vi "KeyboardNudge.vi"(0 "WaveformGraph Refnum":refnum<vi>, 1 "Axis Tune Refnum":refnum<vi>, 3 "Char":i16, 4 "Position (mm) Refnum":refnum<vi>, 5 "Ignore Key Down":bool, 6 "VKey":T2, 7 "PlatMods":T7, 10 "Daxsonics Settings":refnum<vi>, 11 "Pulser":T1, 12 "Inc. Step Size (mm)":dbl=0.5, 13 "Motion Settings":T3={"No Motion?"=FALSE, "Motion System"=enum."MM3000", "Motion Bd ID"=0, "Motion Profile"="", "# Axis"=0, "Reverse Z axis?"=FALSE, "SMAC Axis"=0, "scan pair"=enum."y-(x) scan", "RT fps"=0.0, "Steps per mm"=[], "Motor Parameters"={"velocity ct/s"=[], "accel ct/s^2"=[]}, "One Way Scan"=FALSE, "Reverse One Way Scan"=FALSE, "Global Position (mm)"=[], "Plane"=0, "Distance between\nscan lines (um)"=0.0, "Distance between\nscan planes (um)"=0.0, "number of scan planes"=0, "Total steps in line"=0, "Xtra plane\ndistance  (um)"=0, "Xtra planes "=0, "Add Axis"=FALSE, "overshoot cts"=0, "BKPT Shift"=0, "Scan Start Time (ms)"=0, "ESP VISA"="", "3rd Axis"=1, "GL Ref Out"=refnum, "Galil Address"=""} {"3rd Axis" items=["x", "y", "z", "w"]; "Xtra planes" min=1; "Xtra plane\ndistance  (um)" min=0; "Distance between\nscan planes (um)" format="%.2f"; "Distance between\nscan lines (um)" format="%.2f"; "SMAC Axis" items=["None"=0, "Axis 1"=1, "Axis 2"=2, "Axis 3"=3, "Axis 4"=4, "Axis 5"=5, "Axis 6"=6, "Axis 7"=7, "Axis 8"=8, "Vector Space 1"=17, "Vector Space 2"=18, "Vector Space 3"=19, "Vector Space 4"=20]; "Motion Bd ID" min=1 max=32 step=1}, 14 "UT340 Controls":refnum<vi>, 15 "JSR Simple":refnum<vi>) -> (18 "Z Move?":bool, 19 "Quit":bool)   [LabVIEW 2022 SP3]
uses:
  NI_controller/-NI_MotionRoutines/MotionParameters.ctl
  NI_controller/-NI_MotionRoutines/MotionSys.ctl
  -MotionRoutines/ScanAxis.ctl
  -MotionRoutines/3rdAxis.ctl
  <vilib>/event_ctls.llb/eventvkey.ctl
  Pulsers/Daxsonics/-DaxSubroutines/Dax_Control_Cluster.ctl
  Pulsers/pulser.ctl
  Pulsers/UTEX/Controls/UTEX Controls Simple.ctl
panel:
  # "1-D and 2-D B scan settings"
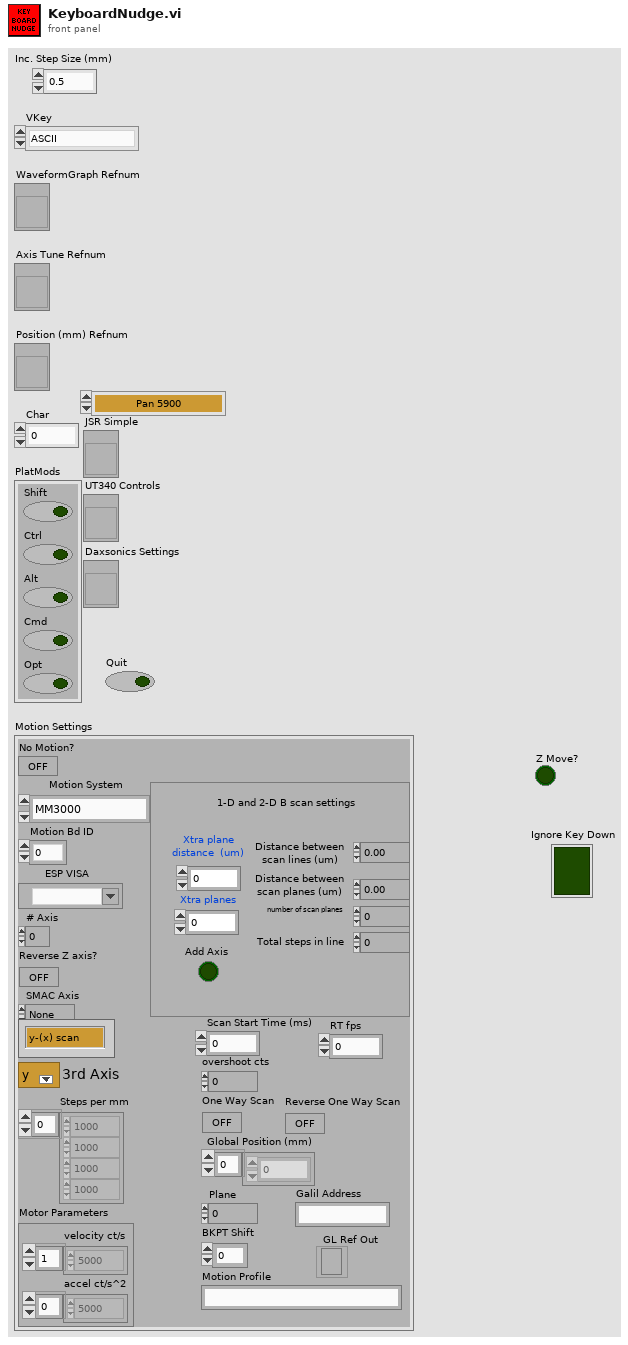
[diagram p1: front panel]
types:
  T1 = typedef "pulser.ctl" = enum16{"Pan 5900", "Daxsonics", "Agilent 33xxx", "UTEX", "JSR", "WMC Mono-Cycle", "No Pulser", "NYU AVTECH", "Tabor W1281A", "Pan 5800", "Unlisted", "Tabor WX2182B"}
  T2 = typedef "eventvkey.ctl" = enum16{"ASCII", "Enter", "Return", "Shift", "Ctrl", "Alt", "Cmd", "Opt", "Caps", "NumLock", "Clear", "Break", "Up", "Down", "Left", "Right", "Insert", "Delete", "Home", "End", "PageUp", "PageDown", "Escape", "Help", "Pause", "ScrollLock", "F1", "F2", "F3", "F4", "F5", "F6", "F7", "F8", "F9", "F10", "F11", "F12", "F13", "F14", "F15", "F16", "F17", "F18", "F19", "F20", "F21", "F22", "F23", "F24", "Play", "VolumeUp", "VolumeDown", "Mute", "Two Byte Char"}
  T3 = typedef "MotionParameters.ctl" = cluster{"No Motion?":bool, "Motion System":T4, "Motion Bd ID":u8, "Motion Profile":string, "# Axis":i8, "Reverse Z axis?":bool, "SMAC Axis":u16, "scan pair":T5, "RT fps":sgl, "Steps per mm":i32[], "Motor Parameters":cluster{"velocity ct/s":dbl[], "accel ct/s^2":dbl[]}, "One Way Scan":bool, "Reverse One Way Scan":bool, "Global Position (mm)":dbl[], "Plane":i32, "Distance between\nscan lines (um)":sgl, "Distance between\nscan planes (um)":sgl, "number of scan planes":i32, "Total steps in line":i32, "Xtra plane\ndistance  (um)":i32, "Xtra planes ":i32, "Add Axis":bool, "overshoot cts":i32, "BKPT Shift":i32, "Scan Start Time (ms)":u32, "ESP VISA":refnum<visa-resource-name>, "3rd Axis":T6, "GL Ref Out":refnum<k7>, "Galil Address":string}
  T4 = typedef "MotionSys.ctl" = enum16{"MM3000", "NI 735x", "Newport ESP", "No Motion Card", "Galil"}
  T5 = typedef "ScanAxis.ctl" = enum16{"y-(x) scan", "x-(y) scan", "z-(x) scan", "z-(y) scan", "y-(z) scan", "x-(z) scan", "w-(x) scan", "w-(y) scan", "w-(z) scan", "x-(w) scan", "y-(w) scan", "z-(w) scan"}
  T6 = typedef "3rdAxis.ctl" = u16
  T7 = cluster{"Shift":bool, "Ctrl":bool, "Alt":bool, "Cmd":bool, "Opt":bool}
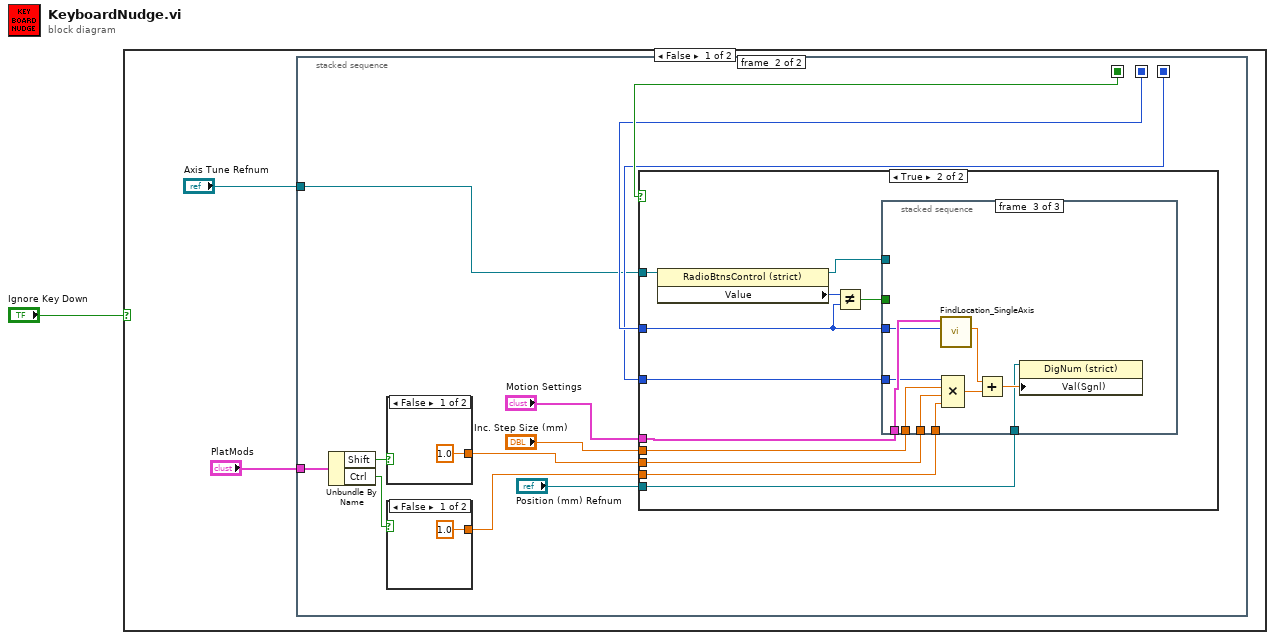
[diagram p0: block diagram]
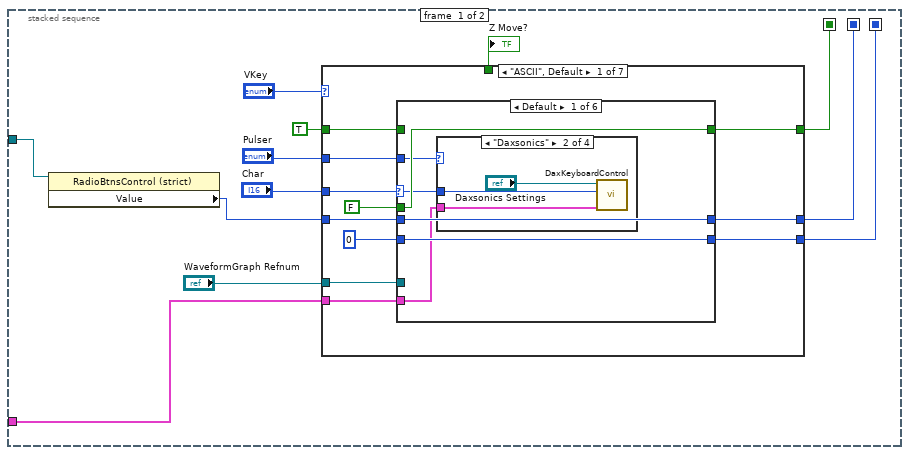
[diagram p2: hidden frame]
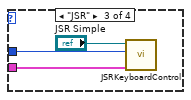
[diagram p4: hidden frame]
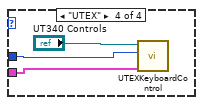
[diagram p5: hidden frame]
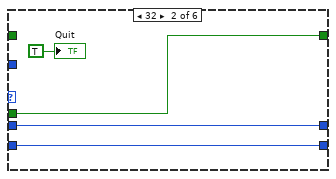
[diagram p6: hidden frame]
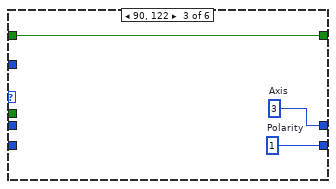
[diagram p7: hidden frame]
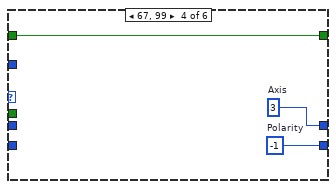
[diagram p8: hidden frame]
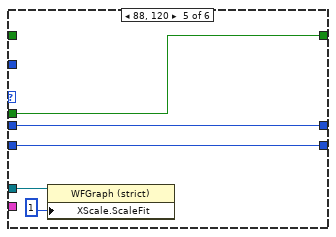
[diagram p9: hidden frame]
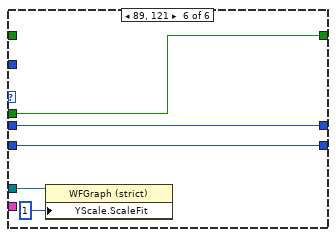
[diagram p10: hidden frame]
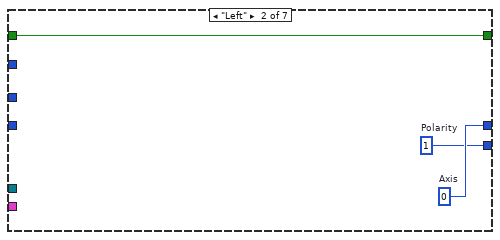
[diagram p11: hidden frame]
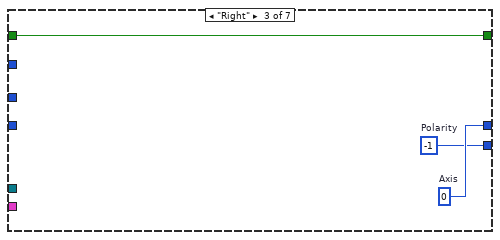
[diagram p12: hidden frame]
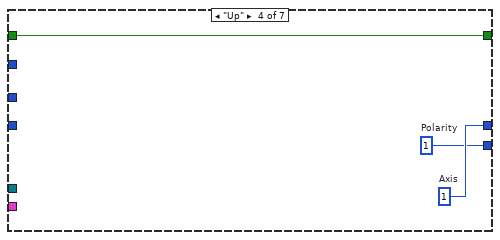
[diagram p13: hidden frame]
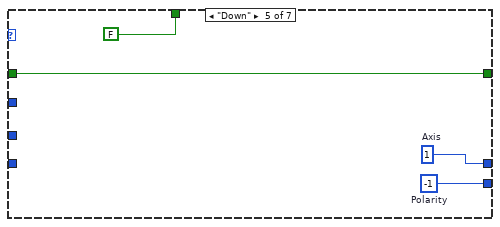
[diagram p14: hidden frame]
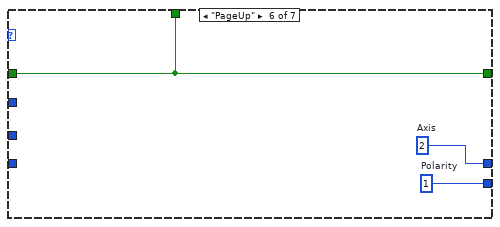
[diagram p15: hidden frame]
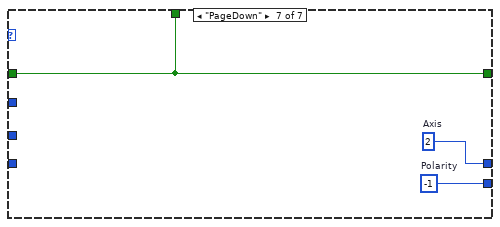
[diagram p16: hidden frame]
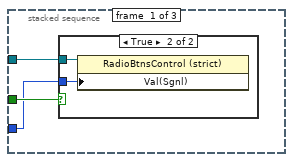
[diagram p18: hidden frame]
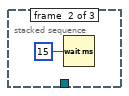
[diagram p20: hidden frame]
diagram:
  n1 = case shown="False" "Ignore Key Down" {
    frame False {
      n2 = stacked-sequence {
        seq-local: [w13 _] -> [_ w83]
        seq-local: [w11 _] -> [_ w84]
        seq-local: [w10 _] -> [_ w85]
        tunnel: "Axis Tune Refnum" -> [w4 w82]
        tunnel: "PlatMods" -> [w6 w81]
        frame #0 {
          n3 = property class="RadioBtnsControl (strict)"(reference=w4) -> ("Value"=w5:enum32{"Axis 1", "Axis 2", "Axis 3", "Axis 4"})  [unwired: 1 in, 2 out]
          n4 = case shown="\"ASCII\", Default" "VKey" {
            tunnel: [w22 w64 w67 w70 w74 w77 w80] -> w11
            tunnel: [w25 w63 w66 w69 w73 w76 w79] -> w13
            tunnel: [w21 w62 w65 w68 w72 w75 w78] -> w10
            tunnel: TRUE -> [w20 w62 w65 w68 w72 w75 w78]
            tunnel: w5 -> [w23 _ _ _ _ _ _]
            tunnel: "Char" -> [w26 _ _ _ _ _ _]
            tunnel: "WaveformGraph Refnum" -> [w18 _ _ _ _ _ _]
            tunnel: [_ _ _ _ FALSE w75 w78] -> w8
            tunnel: w6 -> [w17 _ _ _ _ _ _]
            tunnel: "Pulser" -> [w16 _ _ _ _ _ _]
            frame "ASCII", Default {
              n5 = case shown="Default" w26 {
                selector: w26 -> [w28 _ _ _ _ _]
                tunnel: [w32 w45 w48 w51 w54 w59] -> w25
                tunnel: 0 ("Polarity") -> [w32 w45 _ _ w54 w59]
                tunnel: [w31 w44 w47 w50 w55 w60] -> w22
                tunnel: w23 -> [w31 w44 _ _ w55 w60]
                tunnel: [w30 w43 w46 w49 w53 w58] -> w21
                tunnel: w20 -> [_ _ w46 w49 _ _]
                tunnel: FALSE -> [w30 w43 _ _ w53 w58]
                tunnel: w18 -> [_ _ _ _ w52 w57]
                tunnel: w17 -> [w29 _ _ _ _ _]
                tunnel: w16 -> [w27 _ _ _ _ _]
                frame Default {
                  n6 = case shown="\"Daxsonics\"" w27 {
                    tunnel: w29 -> [_ w35 w37 w39]
                    tunnel: w28 -> [_ w34 w38 w40]
                    frame "Pan 5900", Default {
                    }
                    frame "Daxsonics" {
                      n7 = call "DaxKeyboardControl.vi"("PlatMods"=w35, "Char"=w34, "Daxsonics Settings"="Daxsonics Settings") -> ()  [unwired: 9 in]
                    }
                    frame "JSR" {
                      n8 = call "JSRKeyboardControl.vi"("PlatMods"=w37, "Char"=w38, "JSR Simple"="JSR Simple") -> ()  [unwired: 9 in]
                    }
                    frame "UTEX" {
                      n9 = call "UTEXKeyboardControl.vi"("PlatMods"=w39, "Char"=w40, "UT340 Controls"="UT340 Controls") -> ()  [unwired: 9 in]
                    }
                  }
                }
                frame 32 {
                  "Quit" <- TRUE ("Quit")
                }
                frame 90, 122 {
                  w48 = 1  # Polarity
                  w47 = 3  # Axis
                }
                frame 67, 99 {
                  w51 = -1  # Polarity
                  w50 = 3  # Axis
                }
                frame 88, 120 {
                  n10 = property on="Property Node" class="WFGraph (strict)"(reference=w52, "XScale.ScaleFit"=u8 1 ("X Scale.Scale Fit")) -> ()  [unwired: 1 in, 2 out]
                }
                frame 89, 121 {
                  n11 = property on="Property Node" class="WFGraph (strict)"(reference=w57, "YScale.ScaleFit"=u8 1 ("X Scale.Scale Fit")) -> ()  [unwired: 1 in, 2 out]
                }
              }
            }
            frame "Left" {
              w63 = 1  # Polarity
              w64 = 0  # Axis
            }
            frame "Right" {
              w66 = -1  # Polarity
              w67 = 0  # Axis
            }
            frame "Up" {
              w69 = 1  # Polarity
              w70 = 1  # Axis
            }
            frame "Down" {
              w73 = -1  # Polarity
              w74 = 1  # Axis
            }
            frame "PageUp" {
              w76 = 1  # Polarity
              w77 = 2  # Axis
            }
            frame "PageDown" {
              w79 = -1  # Polarity
              w80 = 2  # Axis
            }
          }
          "Z Move?" <- w8
        }
        frame #1 {
          n12 = Unbundle By Name(w81) -> ("Shift"=w92:bool, "Ctrl"=w87:bool)
          n13 = case shown="False" w92 {
            tunnel: [1.0 0.1] -> w89
            frame False {
            }
            frame True {
            }
          }
          n14 = case shown="False" w87 {
            tunnel: [1.0 0.01] -> w86
            frame False {
            }
            frame True {
            }
          }
          n15 = case shown="True" w85 {
            tunnel: "Inc. Step Size (mm)" -> [_ w103]
            tunnel: w89 -> [_ w102]
            tunnel: w84 -> [_ w100]
            tunnel: "Motion Settings" -> [_ w98]
            tunnel: w86 -> [_ w97]
            tunnel: w83 -> [_ w96]
            tunnel: "Position (mm) Refnum" -> [_ w95]
            tunnel: w82 -> [_ w94]
            frame False {
            }
            frame True {
              n16 = property on="Property Node" class="RadioBtnsControl (strict)"(reference=w94) -> (reference out=w93:refnum<vi>, "Value"=w101:enum32{"Axis 1", "Axis 2", "Axis 3", "Axis 4"})  [unwired: 1 in, 1 out]
              n17 = Not Equal?(x=w101, y=w100) -> (x != y?=w99:bool)
              n18 = stacked-sequence {
                tunnel: w100 -> [w105 _ w111]
                tunnel: w99 -> [w106 _ _]
                tunnel: w96 -> [_ _ w110]
                tunnel: w93 -> [w104 _ _]
                tunnel: w103 -> [_ _ w119]
                tunnel: w102 -> [_ _ w118]
                tunnel: w98 -> [_ _ w114]
                tunnel: w97 -> [_ _ w113]
                tunnel: w95 -> [_ _ w112]
                frame #0 {
                  n19 = case shown="True" w106 {
                    tunnel: w105 -> [_ w108]
                    tunnel: w104 -> [_ w107]
                    frame False {
                    }
                    frame True {
                      n20 = property on="Property Node" class="RadioBtnsControl (strict)"(reference=w107, "Val(Sgnl)"=w108) -> ()  [unwired: 1 in, 2 out]
                    }
                  }
                }
                frame #1 {
                  n21 = Wait (ms)(milliseconds to wait=u32 15) -> ()  [unwired: 1 out]
                }
                frame #2 {
                  n22 = call "FindLocation_SingleAxis.vi"("Axis (0 is X)"=w111, "Motion Settings"=w114) -> ("Position (mm) (Abs)"=w115:dbl)  [unwired: 2 in, 3 out]
                  n23 = Compound Arithmetic op=MULTIPLY(w110, w119, w118, w113) -> (w117:dbl)
                  n24 = Add(x=w115, y=w117) -> (x+y=w116:dbl)
                  n25 = property on="Property Node" class="DigNum (strict)"(reference=w112, "Val(Sgnl)"=w116) -> ()  [unwired: 1 in, 2 out]
                }
              }
            }
          }
        }
      }
    }
    frame True {
    }
  }
